vi "FrequencySet_DDR.vi"(6 "error in":errorcluster, 8 "Did":i32 min=0 max=2 step=1, 9 "VCO Frequency":i32=2400) -> (0 "error out":errorcluster)   [LabVIEW 2011]
doc: "This VI sets the frequency of the DDR PLL.\n\nInputs:\n1. Frequency: Selects the frequency that the DDR PLL will be set to.\n2. Did: The Did value of the DDR frequency."
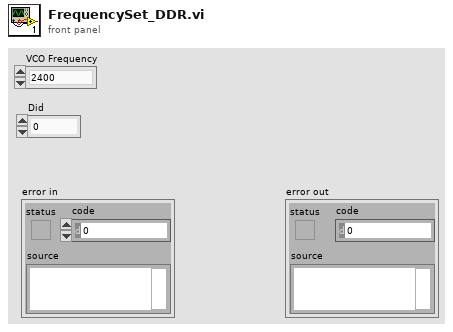
[diagram p1: front panel]
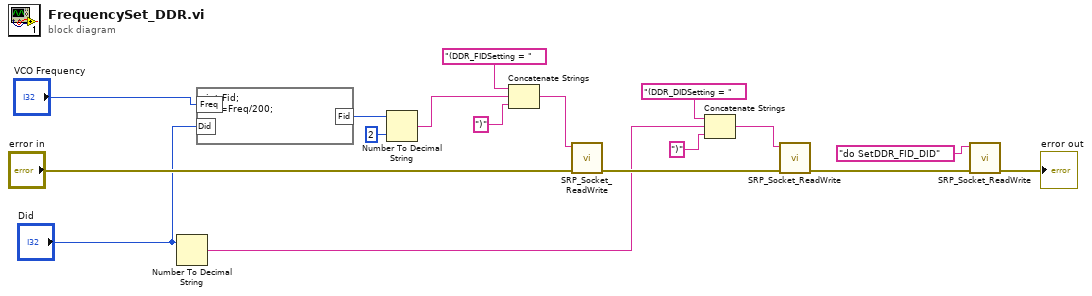
[diagram p0: block diagram]
diagram:
  n1 = Number To Decimal String(number="Did") -> (decimal integer string=w2:string)  [unwired: 1 in]
  n2 = formula code="int Fid;\nFid=Freq/200;"("Freq"="VCO Frequency", "Did"="Did") -> ("Fid"=w8:i32)
  n3 = Number To Decimal String(number=w8, width (-)=i16 2) -> (decimal integer string=w13:string)
  n4 = Concatenate Strings("(DDR_FIDSetting = ", w13, ")") -> (w5:string)
  n5 = call "SRP_Socket_ReadWrite.vi"("error in (no error)"="error in", "Data In"=w5) -> ("error out"=w10:errorcluster)  [unwired: 7 in, 1 out]
  n6 = Concatenate Strings("(DDR_DIDSetting = ", w2, ")") -> (w4:string)
  n7 = call "SRP_Socket_ReadWrite.vi"("error in (no error)"=w10, "Data In"=w4) -> ("error out"=w9:errorcluster)  [unwired: 7 in, 1 out]
  n8 = call "SRP_Socket_ReadWrite.vi"("error in (no error)"=w9, "Data In"="do SetDDR_FID_DID") -> ("error out"=→"error out":errorcluster)  [unwired: 7 in, 1 out]
